vi "Auto - 单工位.vi"() -> ()   [LabVIEW 2020]
uses:
  Global_Variable/A131258.vi
  Global_Variable/Global.vi
  Database/Global1.vi
  <vilib>/addons/database/Connection.llb/DB Tools Open Connec (String).vi
  Libraries/S7/S7.lvlib
  <vilib>/addons/database/NI_Database_API.lvlib
panel:
  in  "Initialize 4":bool
  in  "Initialize 5":bool
  in  "Initialize 3":bool
  in  "Initialize 2":bool
  out "传感器码临时存放":string
  out "初始化":bool[](array[boolean])
  out "磨合台":cluster{dbl[], dbl[]}[](graph)
  in  "判定结果":bool[][](array[boolean])=[[TRUE]]
  in  "STEP":string
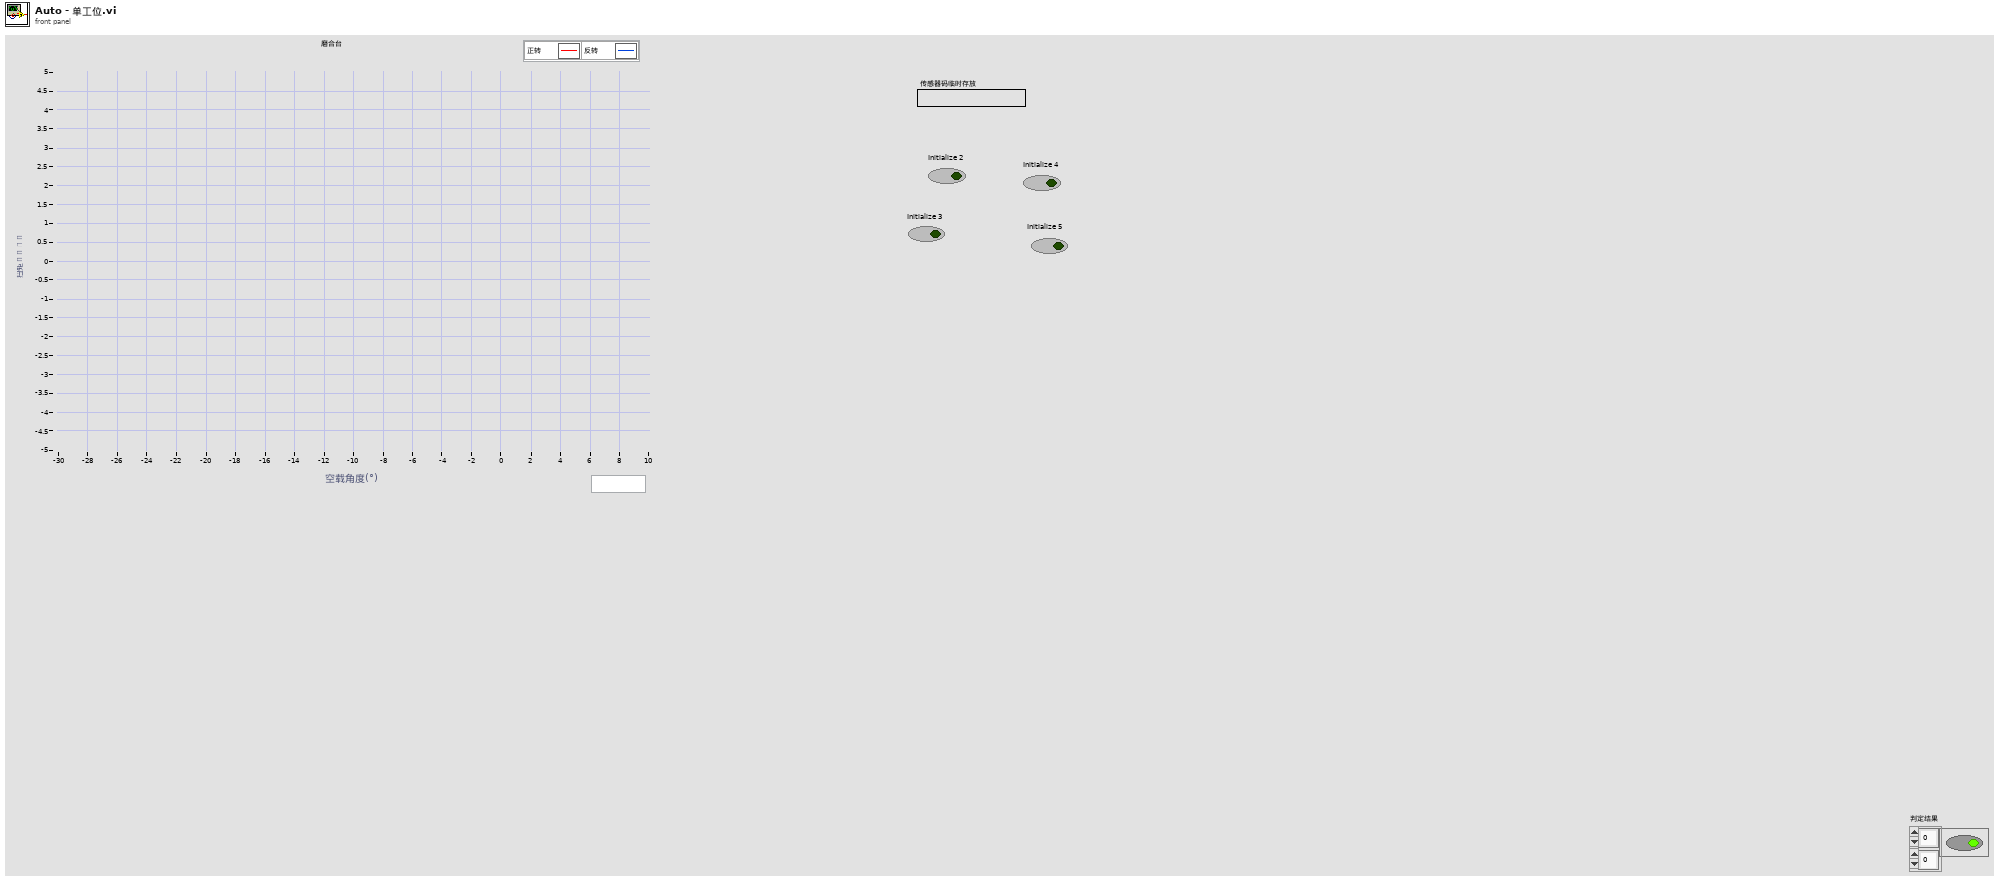
[diagram p1: front panel]
types:
  T1 = cluster{"正转扭矩最大值":cluster{"单位":string, "下限":dbl, "上限":dbl}, "正转扭矩最小值":cluster{"单位":string, "下限":dbl, "上限":dbl}, "正转扭矩波动值":cluster{"单位":string, "下限":dbl, "上限":dbl}, "正转平均扭矩值":cluster{"单位":string, "下限":dbl, "上限":dbl}, "反转扭矩最大值":cluster{"单位":string, "下限":dbl, "上限":dbl}, "反转扭矩最小值":cluster{"单位":string, "下限":dbl, "上限":dbl}, "反转扭矩波动值":cluster{"单位":string, "下限":dbl, "上限":dbl}, "反转扭矩平均值":cluster{"单位":string, "下限":dbl, "上限":dbl}, "正/逆转平均扭矩差":cluster{"单位":string, "下限":dbl, "上限":dbl}}
  T2 = cluster{"正向判定X值":cluster{"单位":string, "下限":dbl, "上限":dbl}, "正向判定Y值":cluster{"单位":string, "下限":dbl, "上限":dbl}, "逆向判定X值":cluster{"单位":string, "下限":dbl, "上限":dbl}, "逆向判定Y值":cluster{"单位":string, "下限":dbl, "上限":dbl}}
  T3 = typedef "NI_Database_API.lvlib/Conn ObjectReference.ctl" = refnum<k1>
  T4 = cluster{"平均扭矩系数":cluster{"单位":string, "正转":dbl, "反转":dbl}, "扭矩波动系数":cluster{"单位":string, "正转":dbl, "反转":dbl}, "空载系数":cluster{"单位":string, "正转":dbl, "反转":dbl}, "零点漂移":cluster{"单位":string, "左":dbl, "右":dbl}}
  T5 = typedef "lveventtype.ctl" = enum32{"Null", "Timeout", "Annotation Menu Selection", "Annotation Menu Selection?", "App Instance Close", "App Instance Close?", "Autoscale Range Change", "Bookmark Info Change", "Cell Edit", "Cell Edit?", "Cursor Grab", "Cursor Grab?", "Cursor Menu Selection", "Cursor Menu Selection?", "Cursor Move", "Cursor Release", "Data Change", "Direction Change", "Display State Change", "Drag Ended", "Drag Enter", "Drag Leave", "Drag Over", "Drag Source Update", "Drag Starting", "Drag Starting?", "Drop", "Exec State Change", "Key Down", "Key Down?", "Key Repeat", "Key Repeat?", "Key Up", "Listbox Double Click", "Menu Activation?", "Menu Selection (App)", "Menu Selection? (App)", "Menu Selection (User)", "Mouse Down", "Mouse Down?", "Mouse Enter", "Mouse Leave", "Mouse Move", "Mouse Up", "Mouse Wheel", "NI Security User Change (App)", "Pane Size", "Panel Close", "Panel Close?", "Panel Resize", "Plot Attribute Change", "Scale Range Change", "Shortcut Menu Activation?", "Shortcut Menu Selection (App)", "Shortcut Menu Selection? (App)", "Shortcut Menu Selection (User)", "Tree Double Click", "Tree Drag", "Tree Drag?", "Tree Drop", "Tree Drop?", "Tree Item Close", "Tree Item Close?", "Tree Item Open", "Tree Item Open?", "User Event", "Value Change"}
  T6 = typedef "LVPoint32TypeDef.ctl" = cluster{"Horizontal":i32, "Vertical":i32}
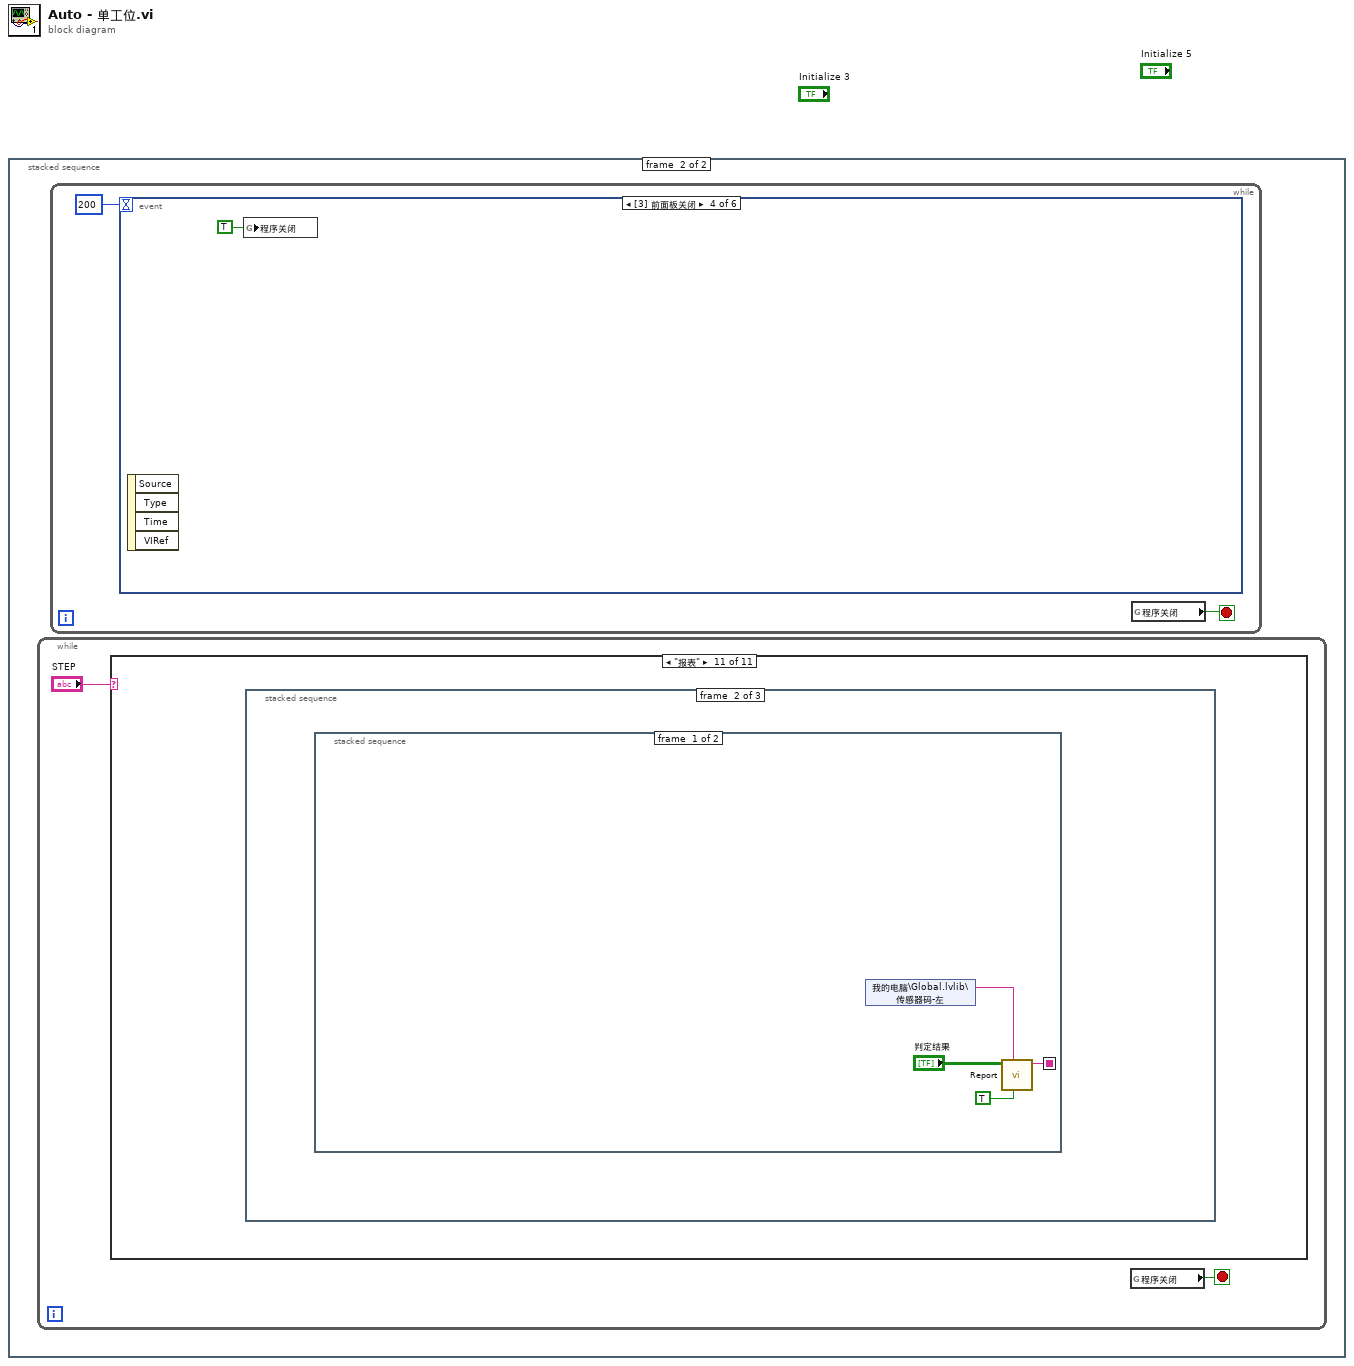
[diagram p0: block diagram]
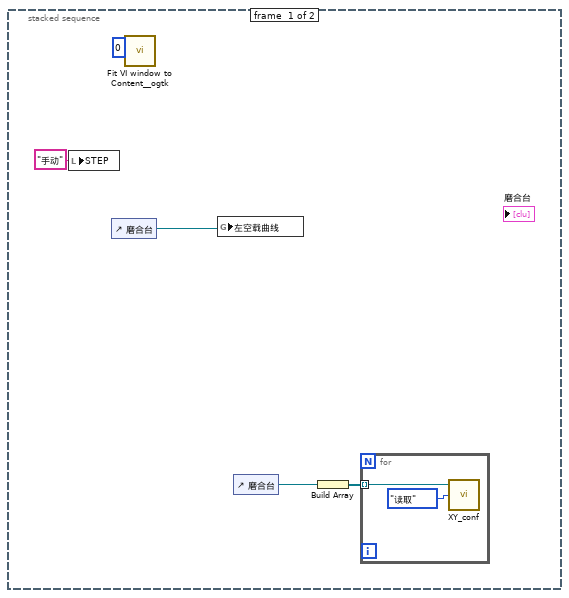
[diagram p2: hidden frame]
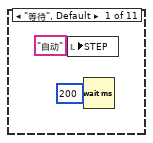
[diagram p3: hidden frame]
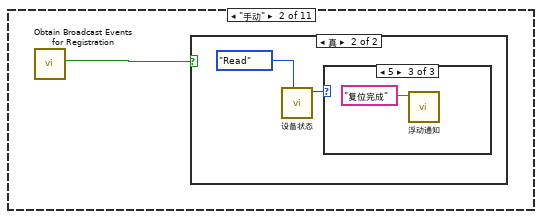
[diagram p4: hidden frame]
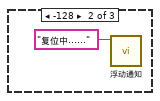
[diagram p7: hidden frame]
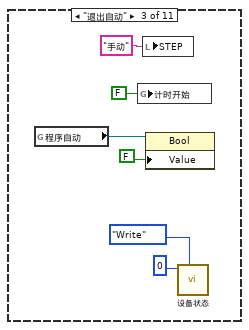
[diagram p8: hidden frame]
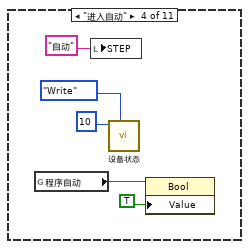
[diagram p9: hidden frame]
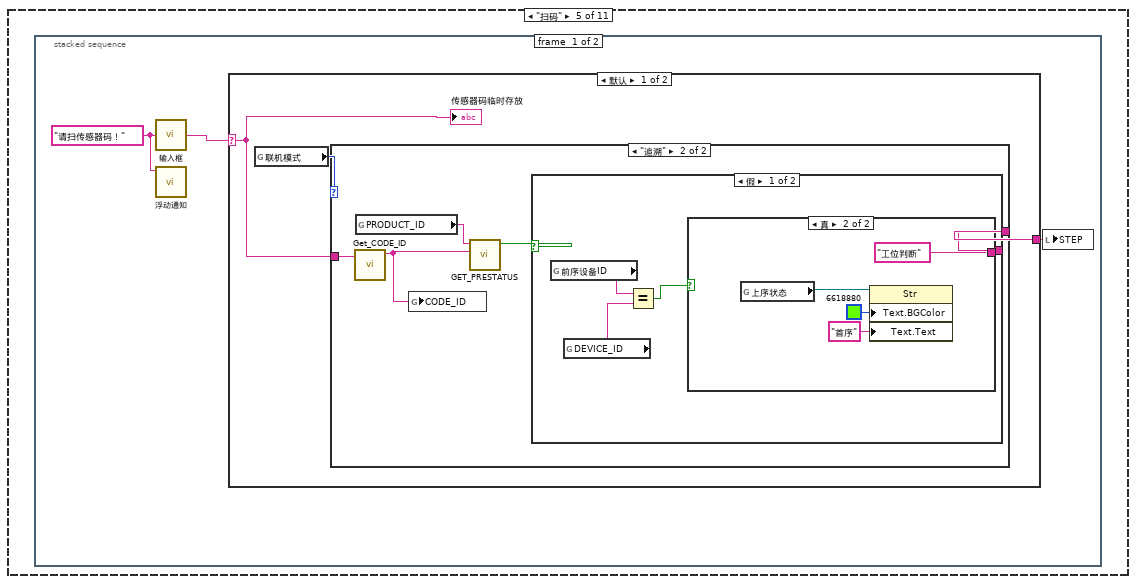
[diagram p10: hidden frame]
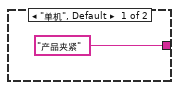
[diagram p11: hidden frame]
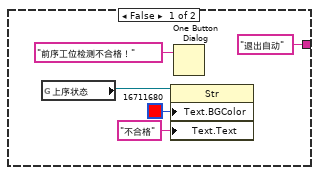
[diagram p12: hidden frame]
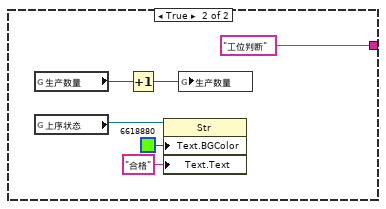
[diagram p13: hidden frame]
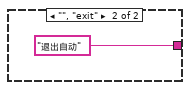
[diagram p14: hidden frame]
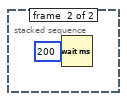
[diagram p15: hidden frame]
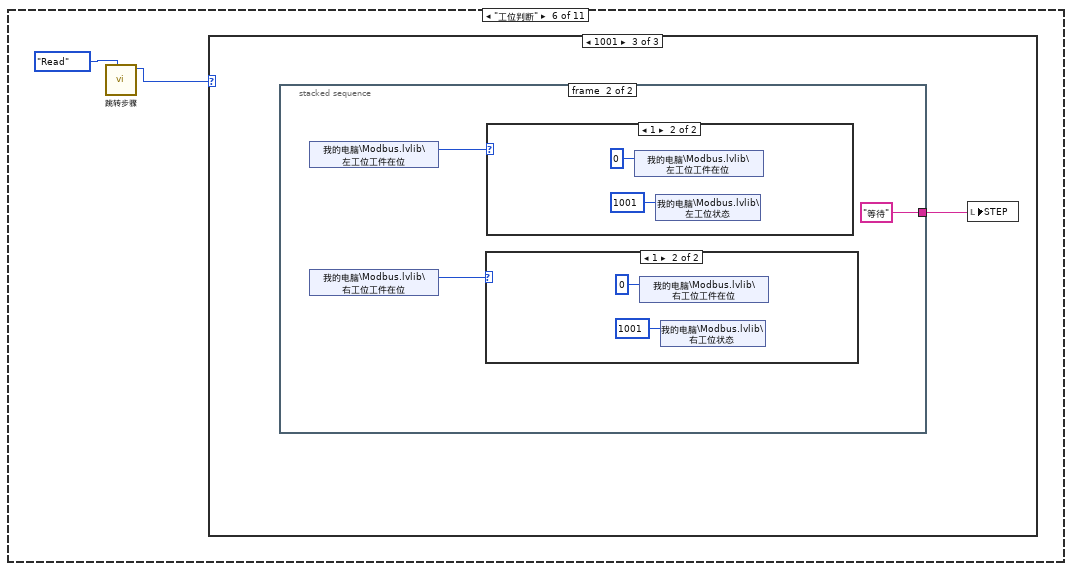
[diagram p16: hidden frame]
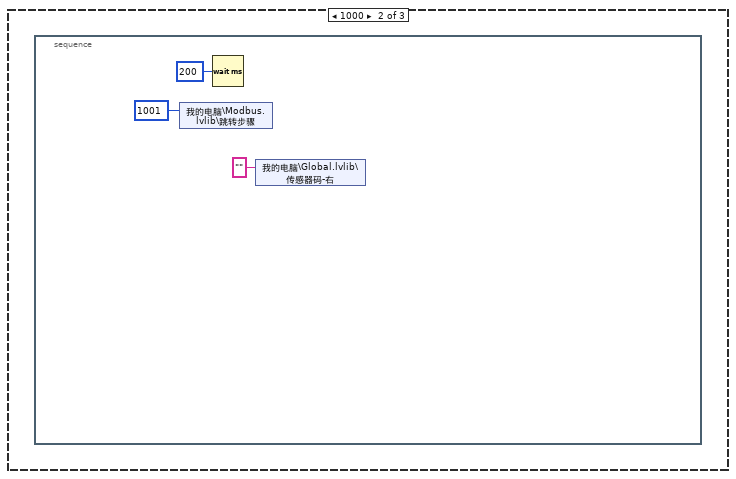
[diagram p18: hidden frame]
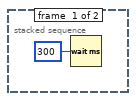
[diagram p19: hidden frame]
diagram:
  n1 = stacked-sequence {
    frame #0 {
      n2 = local write "STEP"("手动" ("STEP")) -> ()
      n3 = control-ref of="磨合台"() -> (w1:refnum<vi>)
      n4 = call <userlib>:"Fit VI window to Content__ogtk.vi"("border spacing (2 px)"=0) -> ()  [unwired: 5 in, 2 out]
      n5 = global write "A131258.vi" "左空载曲线"(w1) -> ()
      n6 = control-ref of="磨合台"() -> (w2:refnum<vi>)
      n7 = Build Array(w2) -> (w3:refnum<vi>[])
      n8 = for {
        tunnel: w3 -> [w6] mode=indexing
        n9 = call "XY_conf.vi"("方式"=enum16{"写入", "读取"}."读取", "XY图引用"=w6) -> ()  [unwired: 3 in, 1 out]
      }
    }
    frame #1 {
      n10 = while {
        stop <- w9 stop-if-true
        n11 = case shown="\"报表\"" "STEP" {
          frame "等待", Default {
            n12 = local write "STEP"("自动" ("STEP")) -> ()
            n13 = Wait (ms)(milliseconds to wait=u32 200 ("等待时间（毫秒）")) -> ()  [unwired: 1 out]
          }
          frame "手动" {
            n14 = call "Obtain Broadcast Events for Registration.vi"() -> ("Already running?"=w12:bool)  [unwired: 9 in, 2 out]
            n15 = case shown="真" w12 {
              frame False {
              }
              frame True {
                n16 = call "设备状态.vi"("枚举"=enum16{"Read", "Write"}."Read") -> ("Status_Read"=w14:i16)  [unwired: 10 in]
                n17 = case shown="5" w14 {
                  frame 0, Default {
                  }
                  frame -128 {
                    n18 = call "浮动通知.vi"("通知内容"="复位中……" ("Status")) -> ()  [unwired: 11 in]
                  }
                  frame 5 {
                    n19 = call "浮动通知.vi"("通知内容"="复位完成" ("Status")) -> ()  [unwired: 11 in]
                  }
                }
              }
            }
          }
          frame "退出自动" {
            n20 = global read "Global.vi" "程序自动"() -> (w18:refnum<vi>)
            n21 = global write "Global.vi" "计时开始"(FALSE ("计时开始")) -> ()
            n22 = local write "STEP"("手动" ("STEP")) -> ()
            n23 = property class="Bool"(reference=w18, "Value"=FALSE) -> ()  [unwired: 1 in, 2 out]
            n24 = call "设备状态.vi"("枚举"=enum16{"Read", "Write"}."Write", "Status_Write"=i16 0) -> ()  [unwired: 9 in, 1 out]
          }
          frame "进入自动" {
            n25 = global read "Global.vi" "程序自动"() -> (w24:refnum<vi>)
            n26 = local write "STEP"("自动" ("STEP")) -> ()
            n27 = call "设备状态.vi"("枚举"=enum16{"Read", "Write"}."Write", "Status_Write"=i16 10) -> ()  [unwired: 9 in, 1 out]
            n28 = property class="Bool"(reference=w24, "Value"=TRUE) -> ()  [unwired: 1 in, 2 out]
          }
          frame "扫码" {
            n29 = stacked-sequence {
              frame #0 {
                w29 = "请扫传感器码！" ("提示信息")
                n30 = call "输入框.vi"("提示信息"=w29) -> ("条形码输出"=w30:string)
                n31 = call "浮动通知.vi"("通知内容"=w29) -> ()  [unwired: 11 in]
                n32 = case shown="默认" w30 {
                  selector: w30 -> [w32 _]
                  tunnel: [w33 "退出自动" ("State(s) in Front (\"\")")] -> w28
                  frame Default {
                    n33 = global read "Global1.vi" "联机模式"() -> (w31:enum16{"单机", "追溯"})
                    n34 = case shown="\"追溯\"" w31 {
                      tunnel: ["产品夹紧" ("State(s) in Front (\"\")") w39] -> w33
                      tunnel: w32 -> [_ w38]
                      frame "单机", Default {
                      }
                      frame "追溯" {
                        n35 = call "Get_CODE_ID.vi"("CODE_MAIN"=w38) -> ("CODE_ID"=w35:string)  [unwired: 10 in]
                        n36 = global read "追溯Global.vi" "PRODUCT_ID"() -> (w37:string)
                        n37 = global write "追溯Global.vi" "CODE_ID"(w35) -> ()
                        n38 = call "GET_PRESTATUS.vi"("CODE_ID"=w35, "PRODUCT_ID"=w37) -> ("OK?"=w36:bool)  [unwired: 8 in, 1 out]
                        n39 = case shown="假" w36 {
                          tunnel: [w43 "工位判断" ("State(s) in Front (\"\")")] -> w39
                          frame False {
                            n40 = global read "追溯Global.vi" "前序设备ID"() -> (w42:string)
                            n41 = global read "追溯Global.vi" "DEVICE_ID"() -> (w41:string)
                            n42 = Equal?(x=w42, y=w41) -> (x = y?=w40:bool)
                            n43 = case shown="真" w40 {
                              tunnel: ["退出自动" ("State(s) in Front (\"\")") "工位判断" ("State(s) in Front (\"\")")] -> w43
                              frame False {
                                n44 = global read "Global.vi" "上序状态"() -> (w46:refnum<vi>)
                                n45 = property class="Str"(reference=w46, "Text.BGColor"=u32 16711680 ("文本.文本颜色:背景色"), "Text.Text"="不合格" ("文本.文本")) -> ()  [unwired: 1 in, 2 out]
                                n46 = One Button Dialog(message="前序工位检测不合格！" ("消息")) -> ()  [unwired: 1 in, 1 out]
                              }
                              frame True {
                                n47 = global read "Global.vi" "上序状态"() -> (w51:refnum<vi>)
                                n48 = property class="Str"(reference=w51, "Text.BGColor"=u32 6618880 ("文本.文本颜色:背景色"), "Text.Text"="首序" ("文本.文本")) -> ()  [unwired: 1 in, 2 out]
                              }
                            }
                          }
                          frame True {
                            n49 = global read "Global.vi" "生产数量"() -> (w56:i32)
                            n50 = global read "Global.vi" "上序状态"() -> (w55:refnum<vi>)
                            n51 = Increment(x=w56) -> (x+1=w57:i32)
                            n52 = property class="Str"(reference=w55, "Text.BGColor"=u32 6618880 ("文本.文本颜色:背景色"), "Text.Text"="合格" ("文本.文本")) -> ()  [unwired: 1 in, 2 out]
                            n53 = global write "Global.vi" "生产数量"(w57) -> ()
                          }
                        }
                      }
                    }
                    "传感器码临时存放" <- w32
                  }
                  frame "", "exit" {
                  }
                }
                n54 = local write "STEP"(w28) -> ()
              }
              frame #1 {
                n55 = Wait (ms)(milliseconds to wait=u32 200 ("等待时间（毫秒）")) -> ()  [unwired: 1 out]
              }
            }
          }
          frame "工位判断" {
            n56 = call "跳转步骤.vi"("枚举"=enum16{"Read", "Write"}."Read") -> ("Status_Read"=w61:i16)  [unwired: 10 in]
            n57 = case shown="1001" w61 {
              frame 0, Default {
              }
              frame 1000 {
                n58 = stacked-sequence {
                  frame #0 {
                    n59 = shared-variable "我的电脑\\Modbus.lvlib\\跳转步骤"(u16 1001 ("跳转步骤")) -> ()  [unwired: 1 in, 1 out]
                    n60 = Wait (ms)(milliseconds to wait=u32 200 ("等待时间（毫秒）")) -> ()  [unwired: 1 out]
                    n61 = shared-variable "我的电脑\\Global.lvlib\\传感器码-右"("" ("工位追溯码")) -> ()  [unwired: 1 in, 1 out]
                  }
                }
              }
              frame 1001 {
                n62 = stacked-sequence {
                  tunnel: [_ "等待" ("STEP")] -> w66
                  frame #0 {
                    n63 = Wait (ms)(milliseconds to wait=u32 300 ("等待时间（毫秒）")) -> ()  [unwired: 1 out]
                  }
                  frame #1 {
                    n64 = shared-variable "我的电脑\\Modbus.lvlib\\左工位工件在位"() -> (w69:u16)  [unwired: 1 in, 1 out]
                    n65 = shared-variable "我的电脑\\Modbus.lvlib\\右工位工件在位"() -> (w70:u16)  [unwired: 1 in, 1 out]
                    n66 = case shown="1" w70 {
                      frame 0, Default {
                      }
                      frame 1 {
                        n67 = shared-variable "我的电脑\\Modbus.lvlib\\右工位工件在位"(u16 0 ("右工位工件在位")) -> ()  [unwired: 1 in, 1 out]
                        n68 = shared-variable "我的电脑\\Modbus.lvlib\\右工位状态"(u16 1001 ("左工位状态")) -> ()  [unwired: 1 in, 1 out]
                      }
                    }
                    n69 = case shown="1" w69 {
                      frame 0, Default {
                      }
                      frame 1 {
                        n70 = shared-variable "我的电脑\\Modbus.lvlib\\左工位工件在位"(u16 0 ("左工位工件在位")) -> ()  [unwired: 1 in, 1 out]
                        n71 = shared-variable "我的电脑\\Modbus.lvlib\\左工位状态"(u16 1001 ("左工位状态")) -> ()  [unwired: 1 in, 1 out]
                      }
                    }
                  }
                }
                n72 = local write "STEP"(w66) -> ()
              }
            }
          }
          frame "初始化" {
            n73 = stacked-sequence {
              frame #0 {
                n74 = global write "Global.vi" "IO_Stop"(TRUE ("IO_Stop")) -> ()
                n75 = global write "Global.vi" "计时开始"(TRUE ("计时开始")) -> ()
                n76 = local write "判定结果"(bool[][] [] ("判定结果")) -> ()
              }
              frame #1 {
                n77 = for {
                  N: 12 -> [_]
                  tunnel: [cluster{dbl[], dbl[]} {[], []}] -> w78 mode=indexing
                }
                n78 = local write "磨合台"(w78) -> ()
              }
              frame #2 {
                n79 = global read "Global.vi" "Result"() -> (w86:refnum<vi>)
                n80 = property class="Tbl"(reference=w86, "Value"=string[][] []) -> (reference out=w87:refnum<vi>, error out=w88:errorcluster)  [unwired: 1 in]
                n81 = property class="Tbl"(reference=w87, error in=w88, "Row Headers[]"=string[] [] ("列首字符串[]")) -> ()  [unwired: 2 out]
                n82 = Initialize Array(TRUE, 12 ("维数大小")) -> (→"初始化":bool[])
              }
              frame #3 {
                n83 = local write "STEP"("自动" ("STEP")) -> ()
              }
            }
          }
          frame "判定" {
            n84 = stacked-sequence {
              frame #0 {
                n85 = global read "A131258.vi" "结果判定参数"() -> (w91:T1)
                n86 = local read "磨合台"() -> (w97:cluster{dbl[], dbl[]}[])
                n87 = global read "Global.vi" "Result"() -> (w98:refnum<vi>)
                n88 = call "复检判定.vi"("Result"=w98, "判定参数"=w91, "XY曲线"=w97) -> ("OK？"=w90:bool)  [unwired: 8 in]
                n89 = case shown="假" w90 {
                  frame False {
                    n90 = shared-variable "我的电脑\\Modbus.lvlib\\左工位生产结果"(u16 2 ("左工位生产结果")) -> ()  [unwired: 1 in, 1 out]
                  }
                  frame True {
                    n91 = shared-variable "我的电脑\\Modbus.lvlib\\左工位生产结果"(u16 1 ("左工位生产结果")) -> ()  [unwired: 1 in, 1 out]
                  }
                }
                n92 = Build Array(TRUE ("元素"), w90) -> (w93:bool[])
                n93 = local read "判定结果"() -> (w95:bool[][])
                n94 = Build Array(w93) -> (w92:bool[][])
                n95 = Build Array (concatenate)(w95, w92) -> (w96:bool[][])
                n96 = local write "判定结果"(w96) -> ()
              }
              frame #1 {
                n97 = local write "STEP"("报表" ("STEP")) -> ()
              }
            }
          }
          frame "自动" {
            n98 = call "设备状态.vi"("枚举"=enum16{"Read", "Write"}."Read") -> ("Status_Read"=w103:i16)  [unwired: 10 in]
            n99 = case shown="110" w103 {
              frame -128 {
                n100 = global write "Global.vi" "计时开始"(FALSE ("计时开始")) -> ()
                n101 = call "浮动通知.vi"("通知内容"="复位中……" ("Status")) -> ()  [unwired: 11 in]
              }
              frame 0, Default {
                n102 = global write "Global.vi" "计时开始"(FALSE ("计时开始")) -> ()
                n103 = call "浮动通知.vi"("通知内容"="手动状态！" ("Status")) -> ()  [unwired: 11 in]
              }
              frame 1 {
                n104 = call "浮动通知.vi"("通知内容"="请复位！" ("Status")) -> ()  [unwired: 11 in]
              }
              frame 5 {
                n105 = call "左工位状态.vi"("枚举"=enum16{"Read", "Write"}."Read") -> ("Status_Read"=w110:i16)  [unwired: 10 in]
                n106 = case shown="1001" w110 {
                  frame 0, Default {
                  }
                  frame 1 {
                  }
                  frame 3 {
                    n107 = shared-variable "我的电脑\\Modbus.lvlib\\空载速度"() -> (w119:sgl)  [unwired: 1 in, 1 out]
                    n108 = for {
                      N: 4 -> [_]
                      tunnel: [cluster{dbl[], dbl[]} {[], []}] -> w116 mode=indexing
                    }
                    n109 = shared-variable "我的电脑\\Global.lvlib\\工位追溯码"("" ("工位追溯码")) -> ()  [unwired: 1 in, 1 out]
                    n110 = Multiply(x=w119, y=sgl 6.0) -> (x*y=w118:sgl)
                    n111 = global write "Global.vi" "空载速度(°/s)"(w118) -> ()
                    n112 = local write "磨合台"(w116) -> ()
                    n113 = global read "Global.vi" "Result"() -> (w114:refnum<vi>)
                    n114 = local write "STEP"("扫码" ("STEP")) -> ()
                    n115 = property class="Tbl"(reference=w114, "Row Headers[]"=string[] [] ("行首字符串[]"), "Value"=string[][] [] ("值")) -> ()  [unwired: 1 in, 2 out]
                  }
                  frame 200 {
                    n116 = stacked-sequence {
                      frame #0 {
                        n117 = shared-variable "我的电脑\\Modbus.lvlib\\左工位生产结果"(u16 0 ("左工位生产结果")) -> ()  [unwired: 1 in, 1 out]
                      }
                      frame #1 {
                        n118 = local read "磨合台"() -> (w123:cluster{dbl[], dbl[]}[])
                        n119 = for {
                          tunnel: [w126] -> w124 mode=indexing
                          tunnel: w123 -> [w125] mode=indexing
                          i -> [w127]
                          n120 = case shown="0" w127 {
                            tunnel: [w128 w129] -> w126
                            tunnel: w125 -> [w128 _]
                            frame Default {
                            }
                            frame 0 {
                              n121 = global read "A131258.vi" "判定框参数"() -> (w134:T2)
                              n122 = Unbundle By Name(w134) -> ("正向判定X值.下限"=w133:dbl, "正向判定X值.上限"=w132:dbl, "正向判定Y值.下限"=w131:dbl, "正向判定Y值.上限"=w130:dbl)
                              n123 = Build Array(w130, w131, w131, w130, w130) -> (w135:dbl[])
                              n124 = Build Array(w132, w132, w133, w133, w132) -> (w136:dbl[])
                              n125 = Bundle(w136, w135) -> (w129:cluster{dbl[], dbl[]})  [unwired: 1 in]
                            }
                          }
                        }
                        n126 = local write "磨合台"(w124) -> ()
                      }
                    }
                  }
                  frame 1001 {
                    n127 = stacked-sequence {
                      frame #0 {
                        n128 = local read "传感器码临时存放"() -> (w137:string)
                        n129 = Wait (ms)(milliseconds to wait=u32 200 ("等待时间（毫秒）")) -> ()  [unwired: 1 out]
                        n130 = shared-variable "我的电脑\\Modbus.lvlib\\左工位状态"(u16 1003 ("左工位状态")) -> ()  [unwired: 1 in, 1 out]
                        n131 = shared-variable "我的电脑\\Global.lvlib\\传感器码-左"(w137) -> ()  [unwired: 1 in, 1 out]
                      }
                      frame #1 {
                        n132 = local write "传感器码临时存放"("" ("传感器码临时存放")) -> ()
                      }
                      frame #2 {
                        n133 = global read "Global1.vi" "联机模式"() -> (w141:enum16{"单机", "追溯"})
                        n134 = case shown="\"追溯\"" w141 {
                          selector: w141 -> [_ w151]
                          frame "单机", Default {
                          }
                          frame "追溯" {
                            n135 = shared-variable "我的电脑\\Global.lvlib\\传感器码-左"() -> (w142:string)  [unwired: 1 in, 1 out]
                            n136 = global read "追溯Global.vi" "PRODUCT_ID"() -> (w150:string)
                            n137 = Concatenate Strings(w142, w150) -> (w148:string)
                            n138 = call "GetSQLstring.vi"("联机模式"=w151) -> ("错误输出"=w147:errorcluster, "连接字符串"=w149:string)  [unwired: 9 in]
                            n139 = Build Array(w148) -> (w143:string[])
                            n140 = call-poly <vilib>:"DB Tools Open Connection.vi"("error in (no error)"=w147, "connection information"=w149) -> ("error out"=w144:errorcluster, "connection reference"=w146:T3)  [unwired: 6 in]
                            n141 = for {
                              tunnel: w143 -> [w158] mode=indexing
                              tunnel: w146 -> [w157]
                              shift-right: [w153] -> w145
                              shift-left: w144 -> [w152]
                              n142 = call <vilib>:"DB Tools Insert Data.vi"("data"=w158, "error in (no error)"=w152, "columns"=string[] ["CODE_SENSOR", "PRODUCT_ID"], "table"="Code", "connection reference"=w157) -> ("error out"=w154:errorcluster)  [unwired: 5 in, 1 out]
                              n143 = case shown="无错误" w154 {
                                selector: w154 -> [w159 w160]
                                tunnel: [w159 w161] -> w153
                                frame No Error {
                                }
                                frame Error {
                                n144 = call <vilib>:"Clear Errors.vi"("error in (no error)"=w160) -> ("error out"=w161:errorcluster)  [unwired: 5 in, 1 out]
                                }
                              }
                            }
                            n145 = call <vilib>:"Simple Error Handler.vi"("error in (no error)"=w145) -> ()  [unwired: 4 in, 5 out]
                          }
                        }
                      }
                    }
                  }
                }
              }
              frame 8 {
                n146 = call "浮动通知.vi"("通知内容"="程序停止！" ("Status")) -> ()  [unwired: 11 in]
              }
              frame 20 {
                n147 = local write "STEP"("扫码" ("STEP")) -> ()
              }
              frame 100 {
                n148 = call "浮动通知.vi"("通知内容"="对花键中！" ("Status")) -> ()  [unwired: 11 in]
              }
              frame 200 {
              }
              frame 110 {
                n149 = call "左工位状态.vi"() -> ("Status_Read"=w165:i16)  [unwired: 11 in]
                n150 = case shown="1" w165 {
                  frame 0, Default {
                  }
                  frame 1 {
                    n151 = local write "STEP"("判定" ("STEP")) -> ()
                  }
                  frame 200 {
                    w167 = TRUE ("Initialize 2")
                    n152 = local write "Initialize 2"(w167) -> ()
                    n153 = local write "Initialize 4"(w167) -> ()
                  }
                  frame 500 {
                    n154 = local read "磨合台"() -> (w169:cluster{dbl[], dbl[]}[])
                    n155 = for {
                      tunnel: w169 -> [w171] mode=indexing
                      tunnel: [w170] -> w168 mode=indexing
                      i -> [w172]
                      n156 = case shown="2" w172 {
                        tunnel: w171 -> [w173 w185]
                        tunnel: [w173 w174] -> w170
                        frame 0, Default {
                        }
                        frame 2 {
                          n157 = global read "Global.vi" "空载速度(°/s)"() -> (w179:dbl)
                          n158 = global read "A131258.vi" "系数"() -> (w188:T4)
                          n159 = local write "Initialize 2"(FALSE ("Initialize 2")) -> ()
                          n160 = Unbundle By Name(w188) -> ("空载系数.正转"=w186:dbl)
                          n161 = case shown="假" "Initialize 2" {
                            tunnel: [w189 0.0] -> w180
                            frame False {
                              n162 = Tick Count (ms)() -> (millisecond timer value=w192:u32)
                              n163 = global read "全局 1.vi" "工位2正向磨合开始时间"() -> (w193:u32)
                              n164 = Subtract(x=w192, y=w193) -> (x-y=w191:u32)
                              n165 = Divide(x=w191, y=u32 1000) -> (x/y=w189:dbl)
                              n166 = global write "全局 1.vi" "工位2正向磨合结束时间"(w189) -> ()
                            }
                            frame True {
                              n167 = Tick Count (ms)() -> (millisecond timer value=w194:u32)
                              n168 = global write "全局 1.vi" "工位2正向磨合开始时间"(w194) -> ()
                            }
                          }
                          n169 = global read "全局1.vi" "左加载"() -> (w187:dbl)
                          n170 = Unbundle(w185) -> (w177:dbl[], w184:dbl[])
                          n171 = Multiply(x=w187, y=w186) -> (x*y=w183:dbl)
                          n172 = Build Array (concatenate)(w184, w183) -> (w175:dbl[])
                          n173 = Multiply(x=w179, y=w180) -> (x*y=w178:dbl)
                          n174 = Build Array (concatenate)(w177, w178) -> (w176:dbl[])
                          n175 = Bundle(w176, w175) -> (w174:cluster{dbl[], dbl[]})  [unwired: 1 in]
                        }
                      }
                    }
                    n176 = local write "磨合台"(w168) -> ()
                  }
                  frame 600 {
                    n177 = local read "磨合台"() -> (w197:cluster{dbl[], dbl[]}[])
                    n178 = for {
                      tunnel: w197 -> [w199] mode=indexing
                      tunnel: [w198] -> w196 mode=indexing
                      i -> [w200]
                      n179 = case shown="2" w200 {
                        tunnel: w199 -> [w201 w213]
                        tunnel: [w201 w203] -> w198
                        frame 0, Default {
                        }
                        frame 2 {
                          n180 = global read "Global.vi" "空载速度(°/s)"() -> (w208:dbl)
                          n181 = global read "A131258.vi" "系数"() -> (w216:T4)
                          n182 = local write "Initialize 4"(FALSE ("Initialize 2")) -> ()
                          n183 = Unbundle By Name(w216) -> ("空载系数.反转"=w214:dbl)
                          n184 = case shown="真" "Initialize 4" {
                            tunnel: [w217 w224] -> w209
                            frame False {
                              n185 = Tick Count (ms)() -> (millisecond timer value=w222:u32)
                              n186 = global read "全局 1.vi" "工位2逆向磨合开始时间"() -> (w223:u32)
                              n187 = global read "全局 1.vi" "工位2正向磨合结束时间"() -> (w219:dbl)
                              n188 = Subtract(x=w222, y=w223) -> (x-y=w221:u32)
                              n189 = Divide(x=w221, y=u32 1000) -> (x/y=w218:dbl)
                              n190 = Subtract(x=w219, y=w218) -> (x-y=w217:dbl)
                            }
                            frame True {
                              n191 = Tick Count (ms)() -> (millisecond timer value=w225:u32)
                              n192 = global write "全局 1.vi" "工位2逆向磨合开始时间"(w225) -> ()
                              n193 = global read "全局 1.vi" "工位2正向磨合结束时间"() -> (w224:dbl)
                            }
                          }
                          n194 = global read "全局1.vi" "左加载"() -> (w215:dbl)
                          n195 = Unbundle(w213) -> (w206:dbl[], w212:dbl[])
                          n196 = Multiply(x=w215, y=w214) -> (x*y=w211:dbl)
                          n197 = Build Array (concatenate)(w212, w211) -> (w204:dbl[])
                          n198 = Multiply(x=w208, y=w209) -> (x*y=w207:dbl)
                          n199 = Build Array (concatenate)(w206, w207) -> (w205:dbl[])
                          n200 = Bundle(w205, w204) -> (w203:cluster{dbl[], dbl[]})  [unwired: 1 in]
                        }
                      }
                    }
                    n201 = local write "磨合台"(w196) -> ()
                  }
                  frame 700 {
                    # "1000"
                    n202 = Wait (ms)(milliseconds to wait=u32 100 ("等待时间（毫秒）")) -> ()  [unwired: 1 out]
                    n203 = call "左工位状态.vi"("枚举"=enum16{"Read", "Write"}."Write", "Status_Write"=i16 1) -> ()  [unwired: 9 in, 1 out]
                  }
                }
              }
              frame 316 {
                n204 = local write "STEP"("判定" ("STEP")) -> ()
              }
              frame 1024 {
                n205 = local write "STEP"("退出自动" ("STEP")) -> ()
              }
            }
          }
          frame "不合格" {
            n206 = local write "STEP"("等待" ("STEP")) -> ()
            n207 = Wait (ms)(milliseconds to wait=u32 100 ("等待时间（毫秒）")) -> ()  [unwired: 1 out]
          }
          frame "报表" {
            n208 = stacked-sequence {
              frame #0 {
                n209 = global write "Global.vi" "计时开始"(FALSE ("计时开始")) -> ()
              }
              frame #1 {
                n210 = stacked-sequence {
                  seq-local: [w235 _] -> [_ w239]
                  frame #0 {
                    n211 = shared-variable "我的电脑\\Global.lvlib\\传感器码-左"() -> (w234:string)  [unwired: 1 in, 1 out]
                    n212 = call "Report.vi"("文件重命名"=TRUE, "文件名称"=w234, "检测结果"="判定结果") -> ("PRODUCT_VAULE"=w235:string)  [unwired: 7 in, 1 out]
                  }
                  frame #1 {
                    n213 = global read "Global1.vi" "联机模式"() -> (w238:enum16{"单机", "追溯"})
                    n214 = case shown="\"追溯\"" w238 {
                      tunnel: w239 -> [_ w240]
                      frame "单机", Default {
                      }
                      frame "追溯" {
                        n215 = global read "Global.vi" "Result"() -> (w245:refnum<vi>)
                        n216 = property class="Tbl"(reference=w245) -> (reference out=w244:refnum<vi>, "Row Headers[]"=w242:string[])  [unwired: 1 in, 1 out]
                        n217 = property class="Tbl"(reference=w244) -> ("Value"=w243:string[][])  [unwired: 1 in, 2 out]
                        n218 = for {
                          tunnel: w243 -> [w251] mode=indexing
                          tunnel: w242 -> [w252] mode=indexing
                          tunnel: [w249] -> w241 mode=indexing if=w250
                          n219 = Index Array(array=w251) -> (element=w253:string)  [unwired: 1 in]
                          n220 = Build Array (concatenate)(w252, w251) -> (w249:string[])
                          n221 = case shown="\"\"" w253 {
                            tunnel: [TRUE FALSE] -> w250
                            frame Default {
                            }
                            frame "" {
                            }
                          }
                        }
                        n222 = global read "追溯Global.vi" "DEVICE_ID"() -> (w247:string)
                        n223 = global read "追溯Global.vi" "CODE_ID"() -> (w246:string)
                        n224 = global read "追溯Global.vi" "USER_ID"() -> (w248:string)
                        n225 = call "UPRESULT.vi"("DEVICE_ID"=w247, "USER_ID"=w248, "CODE_ID"=w246, "RESULT_VALUE"=w240) -> ()  [unwired: 11 in, 1 out]
                        n226 = call "UPTEST.vi"("Result"=w241, "CODE_ID"=w246, "DEVICE_ID"=w247) -> ()  [unwired: 6 in, 1 out]
                      }
                    }
                  }
                }
              }
              frame #2 {
                n227 = local write "STEP"("进入自动" ("STEP")) -> ()
              }
            }
          }
        }
        n228 = global read "Global.vi" "程序关闭"() -> (w9:bool)
      }
      n229 = while {
        stop <- w257 stop-if-true
        n230 = event shown="[3] 前面板关闭" {
          selector: _ -> [_ _ _ _ _ _]
          dyn-events: _ -> [_ _ _ _ _ _]
          timeout: 200 -> [_ _ _ _ _ _]
          event Timeout {
            n231 = event-data() -> ()  [unwired: 1 in, 3 out]
            n232 = call "Obtain Broadcast Events for Registration.vi"() -> ("Already running?"=w259:bool)  [unwired: 9 in, 2 out]
            n233 = case shown="真" w259 {
              frame False {
                n234 = local write "STEP"("手动" ("STEP")) -> ()
              }
              frame True {
                n235 = call "错误代码.vi"() -> ("Status_Read"=w261:u32)  [unwired: 11 in]
                n236 = feedback #1() -> (w271:u32)  [unwired: 1 in]
                n237 = feedback-in #1(w261) -> ()
                n238 = case shown="0" w261 {
                  frame 0 {
                    n239 = global read "Global.vi" "报警图标"() -> (w272:refnum<vi>)
                    n240 = property class="Bool"(reference=w272, "Visible"=FALSE ("可见")) -> ()  [unwired: 1 in, 2 out]
                  }
                  frame 1, Default {
                    n241 = global read "Global.vi" "报警图标"() -> (w275:refnum<vi>)
                    n242 = property class="Bool"(reference=w275, "Visible"=TRUE ("可见")) -> ()  [unwired: 1 in, 2 out]
                  }
                }
                n243 = Greater Or Equal?(x=w261, y=i16 5000) -> (x >= y?=w269:bool)
                n244 = Less?(x=w261, y=i16 5200) -> (x < y?=w270:bool)
                n245 = Equal?(x=w261, y=w271) -> (x = y?=w268:bool)
                n246 = global read "Global.vi" "报警图标"() -> (w263:refnum<vi>)
                n247 = And(x=w269, y=w270) -> (x .and. y?=w262:bool)
                n248 = property class="Bool"(reference=w263, "Value"=w262) -> ()  [unwired: 1 in, 2 out]
                n249 = Bundle By Name(cluster=errorcluster {"status"=FALSE, "code"=0, "source"=""} ("错误常量"), "status"=w262, "code"=w261) -> (w267:errorcluster)
                n250 = case shown="假" w268 {
                  tunnel: w267 -> [w276 _]
                  frame False {
                    n251 = call "报警处理.vi"("错误常量"=w276) -> ()  [unwired: 9 in, 2 out]
                  }
                  frame True {
                  }
                }
              }
            }
          }
          event Menu Selection (User) {
            n252 = event-data() -> ("ItemTag"=w277:string)  [unwired: 1 in, 2 out]
            n253 = case shown="\"假\", 默认" w277 {
              frame "假", Default {
              }
              frame "真" {
              }
            }
          }
          event "磨合台": Scale Range Change {
            n254 = event-data() -> ("CtlRef"=w278:refnum<vi>)  [unwired: 1 in]
            n255 = call "XY_conf.vi"("方式"=enum16{"写入", "读取"}."写入", "XY图引用"=w278) -> ()  [unwired: 3 in, 1 out]
          }
          event Panel Close {
            n256 = event-data() -> ()  [unwired: 1 in, 4 out]
            n257 = global write "Global.vi" "程序关闭"(TRUE ("程序关闭")) -> ()
          }
          event "磨合台": Mouse Enter; "磨合台": Mouse Leave; "磨合台": Cursor Move {
            n258 = event-data() -> ("CtlRef"=w283:refnum<vi>, "Type"=w281:T5)  [unwired: 1 in]
            n259 = call "CursorShow.vi"("nameShow"=TRUE, "Type"=w281, "Graph"=w283) -> ()  [unwired: 7 in, 2 out]
          }
          event "磨合台": Mouse Down {
            n260 = event-data() -> ("CtlRef"=w288:refnum<vi>, "Coords"=w287:T6, "Type"=w285:T5)  [unwired: 1 in]
            n261 = invoke class="XYGraph (严格)" method="Map Coords To XY"(reference=w288, "Coords"=w287) -> (reference out=w286:refnum<vi>, "XY"=w284:cluster{"X":dbl, "Y":dbl})  [unwired: 5 in, 5 out]
            n262 = call "CursorShow.vi"("游标.游标位置"=w284, "Type"=w285, "Graph"=w286) -> ()  [unwired: 7 in, 2 out]
          }
        }
        n263 = global read "Global.vi" "程序关闭"() -> (w257:bool)
      }
    }
  }
